vi "InitCSMs.vi"(7 "Enable building lvlibp?":bool, 8 "error in":errorcluster, 11 "testcase-CSMStatus in":refnum<class "testcase-CSMBroadcast.lvclass">) -> (0 "error out":errorcluster, 3 "testcase-CSMStatus out":refnum<class "testcase-CSMBroadcast.lvclass">)   [LabVIEW 2017, in "testcase-CSMBroadcast.lvclass"]
uses:
  testcase-CSMBroadcast.lvclass
  CSM/Normal-CSM.vi
  CSM/Chain1.vi
  CSM/Chain2.vi
  CSM/Chain3.vi
  <vilib>/AppBuilder/AB_API_Simple/Build (path).vi
  CSM/CSM-Testcase.lvlib
  src/user.lib/_NEVSTOP/Communicable State Machine(CSM)/Communicable State Machine.lvlib
  <vilib>/AppBuilder/AB_API_Simple/NI_App_Builder_API.lvlib
panel:
  out "Waited (ms)":u32
  out "CSMs Left":string[](array[string])
  out "CSMs":string[](array[string])
  out "Generated files":path[](array[path])
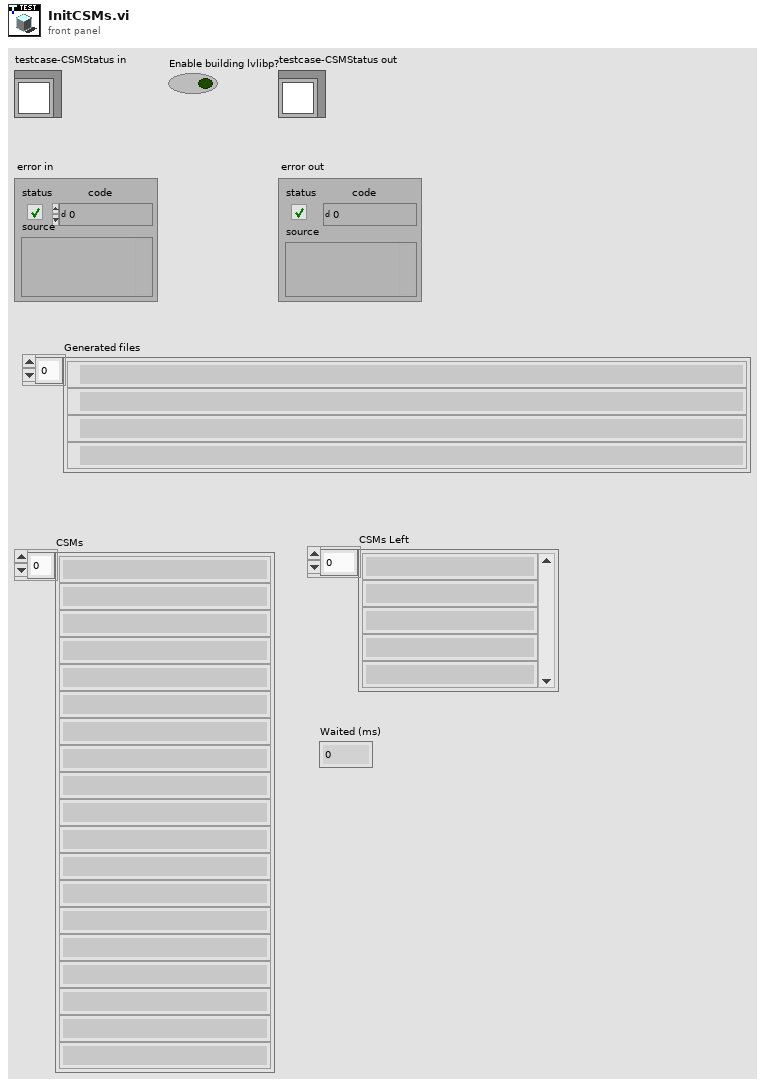
[diagram p1: front panel]
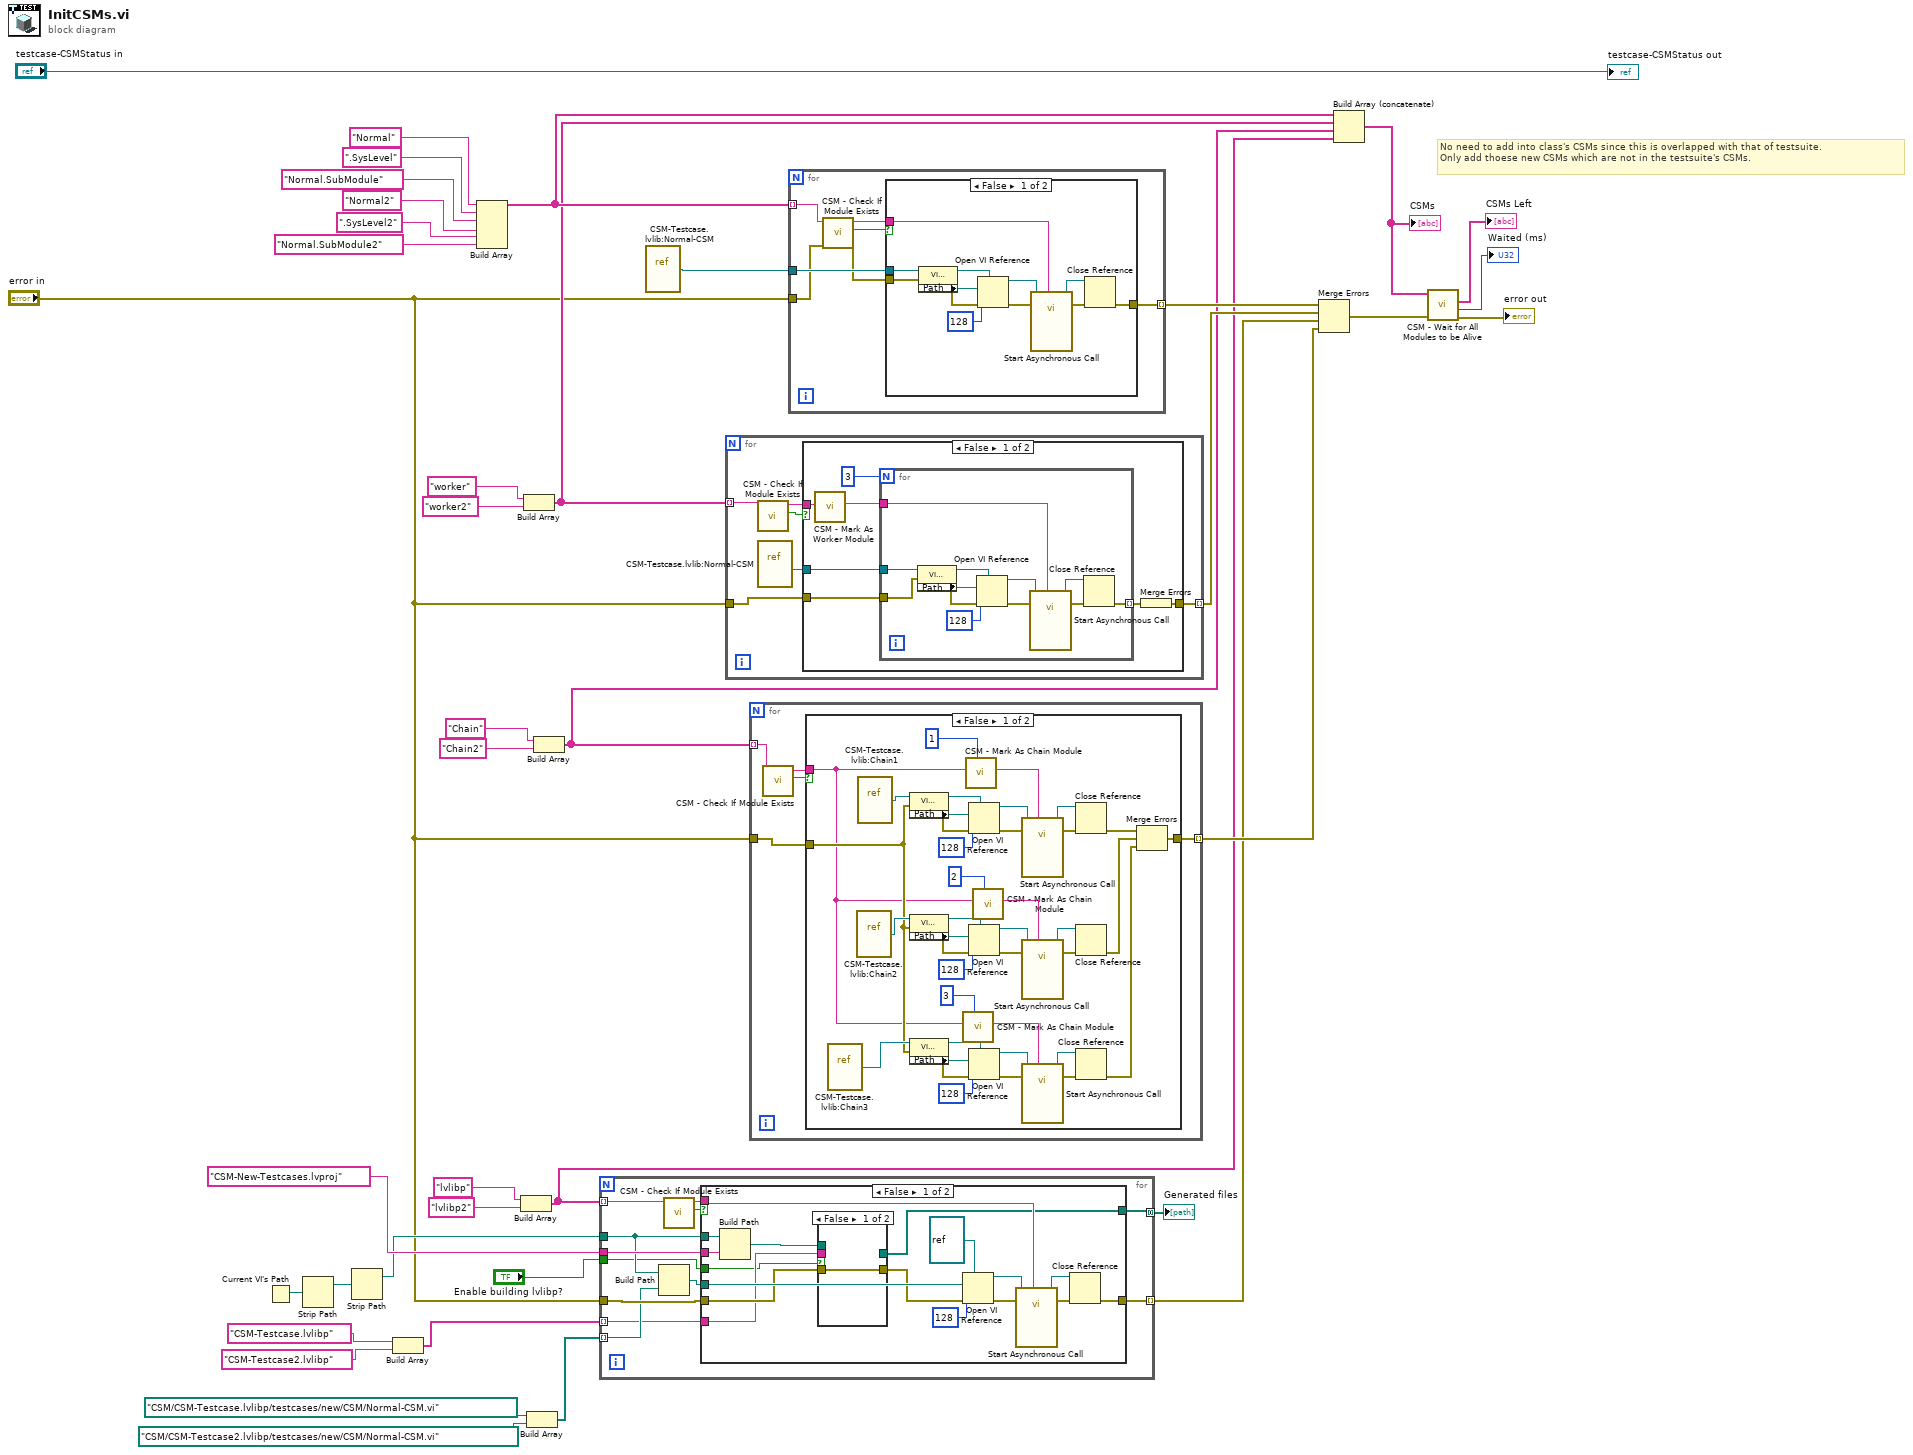
[diagram p0: block diagram]
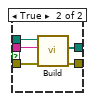
[diagram p2: hidden frame]
diagram:
  # "No need to add into class's CSMs since this is overlapped with that of testsuite.\nOnly add thoese new CSMs which are not in the testsuite's CSMs."
  n1 = Current VI's Path() -> (path=w36:path)
  n2 = Strip Path(path=w36) -> (stripped path=w37:path)  [unwired: 1 out]
  n3 = Strip Path(path=w37) -> (stripped path=w38:path)  [unwired: 1 out]
  n4 = Build Array("CSM-Testcase.lvlibp" ("Name of build specification (if empty: build all)"), "CSM-Testcase2.lvlibp" ("Name of build specification (if empty: build all)")) -> (w10:string[])
  n5 = Build Array("Normal" ("Name (\"\" to Use UUID)"), ".SysLevel" ("Name (\"\" to Use UUID)"), "Normal.SubModule" ("Name (\"\" to Use UUID)"), "Normal2" ("Name (\"\" to Use UUID)"), ".SysLevel2" ("Name (\"\" to Use UUID)"), "Normal.SubModule2" ("Name (\"\" to Use UUID)")) -> (w32:string[])
  n6 = Build Array("lvlibp" ("Name (\"\" to Use UUID)"), "lvlibp2" ("Name (\"\" to Use UUID)")) -> (w16:string[])
  n7 = Build Array("worker" ("Name (\"\" to Use UUID)"), "worker2" ("Name (\"\" to Use UUID)")) -> (w22:string[])
  n8 = Build Array(path "CSM/CSM-Testcase.lvlibp/testcases/new/CSM/Normal-CSM.vi" ("vi path"), path "CSM/CSM-Testcase2.lvlibp/testcases/new/CSM/Normal-CSM.vi" ("vi path")) -> (w13:path[])
  n9 = Build Array("Chain" ("Name (\"\" to Use UUID)"), "Chain2" ("Name (\"\" to Use UUID)")) -> (w19:string[])
  n10 = for {
    tunnel: "CSM-New-Testcases.lvproj" ("name or relative path") -> [w50]
    tunnel: w38 -> [w45]
    tunnel: w16 -> [w47] mode=indexing
    tunnel: w13 -> [w46] mode=indexing
    tunnel: w10 -> [w43] mode=indexing
    tunnel: [w42] -> w9 mode=concatenating
    tunnel: "Enable building lvlibp?" -> [w41]
    tunnel: "error in" -> [w51]
    tunnel: [w49] -> w35 mode=indexing
    n11 = Build Path(base path=w45, name or relative path=w46) -> (appended path=w44:path)
    n12 = call "CSM - Check If Module Exists.vi"("CSM Name"=w47) -> ("Exist?"=w52:bool, "CSM Name (Dup)"=w48:string)  [unwired: 8 in, 1 out]
    n13 = case shown="False" w52 {
      tunnel: [w69 w76] -> w49
      tunnel: w44 -> [w62 _]
      tunnel: w45 -> [w61 _]
      tunnel: w50 -> [w59 _]
      tunnel: w48 -> [w58 _]
      tunnel: w51 -> [w57 w76]
      tunnel: w43 -> [w55 _]
      tunnel: [w54 _] -> w42
      tunnel: w41 -> [w53 _]
      frame False {
        n14 = Build Path(base path=w61, name or relative path=w59) -> (appended path=w60:path)
        n15 = case shown="False" w53 {
          tunnel: w60 -> [_ w75]
          tunnel: w57 -> [w70 w74]
          tunnel: [w70 w73] -> w56
          tunnel: w55 -> [_ w72]
          tunnel: [_ w71] -> w54
          frame False {
          }
          frame True {
            n16 = call-poly <vilib>:"Build.vi"("error in (no error)"=w74, "Name of build specification (if empty: build all)"=w72, "Path to project"=w75) -> ("error out"=w73:errorcluster, "Generated files"=w71:path[])  [unwired: 7 in]
          }
        }
        n17 = Open VI Reference(type specifier VI Refnum (for type only)=refnum<vi> refnum ("reference out"), vi path=w62, options=128, error in (no error)=w56) -> (vi reference=w65:refnum<vi>, error out=w67:errorcluster)  [unwired: 2 in]
        n18 = call-by-ref "Start Asynchronous Call"(reference=w65, error in=w67, "Name (\"\" to Use UUID)"=w58) -> (reference out=w64:refnum<vi>, error out=w66:errorcluster)  [unwired: 11 in]
        n19 = Close Reference(reference=w64, error in (no error)=w66) -> (error out=w69:errorcluster)
      }
      frame True {
      }
    }
  }
  "Generated files" <- w9
  n20 = vi-ref "CSM-Testcase.lvlib:Normal-CSM.vi"() -> (w28:refnum<vi>)
  n21 = for {
    tunnel: w22 -> [w77] mode=indexing
    tunnel: "error in" -> [w82]
    tunnel: [w79] -> w34 mode=indexing
    n22 = call "CSM - Check If Module Exists.vi"("CSM Name"=w77) -> ("Exist?"=w81:bool, "CSM Name (Dup)"=w80:string)  [unwired: 8 in, 1 out]
    n23 = vi-ref "CSM-Testcase.lvlib:Normal-CSM.vi"() -> (w78:refnum<vi>)
    n24 = case shown="False" w81 {
      tunnel: w78 -> [w89 _]
      tunnel: [w83 w102] -> w79
      tunnel: w82 -> [w85 w102]
      tunnel: w80 -> [w84 _]
      frame False {
        n25 = call "CSM - Mark As Worker Module.vi"("CSM Name"=w84) -> ("CSM Name (Marked As Worker)"=w86:string)  [unwired: 9 in]
        n26 = for {
          N: 3 -> [_]
          tunnel: w89 -> [w93]
          tunnel: w86 -> [w92]
          tunnel: [w91] -> w87 mode=indexing
          tunnel: w85 -> [w90]
          n27 = property class="VI (strict)"(reference=w93, error in=w90) -> (reference out=w99:refnum<vi>, error out=w97:errorcluster, "Path"=w96:path)
          n28 = Open VI Reference(type specifier VI Refnum (for type only)=w99, vi path=w96, options=128, error in (no error)=w97) -> (vi reference=w95:refnum<vi>, error out=w100:errorcluster)  [unwired: 2 in]
          n29 = call-by-ref "Start Asynchronous Call"(reference=w95, error in=w100, "Name (\"\" to Use UUID)"=w92) -> (reference out=w94:refnum<vi>, error out=w98:errorcluster)  [unwired: 11 in]
          n30 = Close Reference(reference=w94, error in (no error)=w98) -> (error out=w91:errorcluster)
        }
        n31 = Merge Errors(w87) -> (w83:errorcluster)
      }
      frame True {
      }
    }
  }
  n32 = for {
    tunnel: w19 -> [w103] mode=indexing
    tunnel: "error in" -> [w107]
    tunnel: [w105] -> w40 mode=indexing
    n33 = call "CSM - Check If Module Exists.vi"("CSM Name"=w103) -> ("Exist?"=w106:bool, "CSM Name (Dup)"=w104:string)  [unwired: 8 in, 1 out]
    n34 = case shown="False" w106 {
      tunnel: [w110 w147] -> w105
      tunnel: w107 -> [w109 w147]
      tunnel: w104 -> [w108 _]
      frame False {
        n35 = vi-ref "CSM-Testcase.lvlib:Chain3.vi"() -> (w128:refnum<vi>)
        n36 = vi-ref "CSM-Testcase.lvlib:Chain2.vi"() -> (w129:refnum<vi>)
        n37 = vi-ref "CSM-Testcase.lvlib:Chain1.vi"() -> (w146:refnum<vi>)
        n38 = property class="VI (strict)"(reference=w146, error in=w109) -> (reference out=w143:refnum<vi>, error out=w141:errorcluster, "Path"=w140:path)
        n39 = property class="VI (strict)"(reference=w129, error in=w109) -> (reference out=w132:refnum<vi>, error out=w134:errorcluster, "Path"=w135:path)
        n40 = property class="VI (strict)"(reference=w128, error in=w109) -> (reference out=w125:refnum<vi>, error out=w123:errorcluster, "Path"=w122:path)
        n41 = call "CSM - Mark As Chain Module.vi"("Order"=3, "CSM Name"=w108) -> ("CSM Name (Marked As Chain)"=w116:string)  [unwired: 8 in]
        n42 = call "CSM - Mark As Chain Module.vi"("Order"=1, "CSM Name"=w108) -> ("CSM Name (Marked As Chain)"=w114:string)  [unwired: 8 in]
        n43 = Open VI Reference(type specifier VI Refnum (for type only)=w143, vi path=w140, options=128, error in (no error)=w141) -> (vi reference=w139:refnum<vi>, error out=w144:errorcluster)  [unwired: 2 in]
        n44 = Open VI Reference(type specifier VI Refnum (for type only)=w132, vi path=w135, options=128, error in (no error)=w134) -> (vi reference=w136:refnum<vi>, error out=w131:errorcluster)  [unwired: 2 in]
        n45 = Open VI Reference(type specifier VI Refnum (for type only)=w125, vi path=w122, options=128, error in (no error)=w123) -> (vi reference=w121:refnum<vi>, error out=w126:errorcluster)  [unwired: 2 in]
        n46 = call "CSM - Mark As Chain Module.vi"("Order"=2, "CSM Name"=w108) -> ("CSM Name (Marked As Chain)"=w115:string)  [unwired: 8 in]
        n47 = call-by-ref "Start Asynchronous Call"(reference=w139, error in=w144, "Name (\"\" to Use UUID)"=w114) -> (reference out=w138:refnum<vi>, error out=w142:errorcluster)  [unwired: 11 in]
        n48 = call-by-ref "Start Asynchronous Call"(reference=w136, error in=w131, "Name (\"\" to Use UUID)"=w115) -> (reference out=w137:refnum<vi>, error out=w133:errorcluster)  [unwired: 11 in]
        n49 = call-by-ref "Start Asynchronous Call"(reference=w121, error in=w126, "Name (\"\" to Use UUID)"=w116) -> (reference out=w120:refnum<vi>, error out=w124:errorcluster)  [unwired: 11 in]
        n50 = Close Reference(reference=w138, error in (no error)=w142) -> (error out=w119:errorcluster)
        n51 = Close Reference(reference=w137, error in (no error)=w133) -> (error out=w118:errorcluster)
        n52 = Close Reference(reference=w120, error in (no error)=w124) -> (error out=w117:errorcluster)
        n53 = Merge Errors(w119, w118, w117) -> (w110:errorcluster)
      }
      frame True {
      }
    }
  }
  n54 = for {
    tunnel: w28 -> [w154]
    tunnel: w32 -> [w150] mode=indexing
    tunnel: [w153] -> w33 mode=indexing
    tunnel: "error in" -> [w152]
    n55 = call "CSM - Check If Module Exists.vi"("Error In"=w152, "CSM Name"=w150) -> ("error out"=w151:errorcluster, "Exist?"=w148:bool, "CSM Name (Dup)"=w149:string)  [unwired: 7 in]
    n56 = case shown="False" w148 {
      tunnel: w154 -> [w158 _]
      tunnel: [w157 w167] -> w153
      tunnel: w151 -> [w156 w167]
      tunnel: w149 -> [w155 _]
      frame False {
        n57 = property class="VI (strict)"(reference=w158, error in=w156) -> (reference out=w164:refnum<vi>, error out=w162:errorcluster, "Path"=w161:path)
        n58 = Open VI Reference(type specifier VI Refnum (for type only)=w164, vi path=w161, options=128, error in (no error)=w162) -> (vi reference=w160:refnum<vi>, error out=w165:errorcluster)  [unwired: 2 in]
        n59 = call-by-ref "Start Asynchronous Call"(reference=w160, error in=w165, "Name (\"\" to Use UUID)"=w155) -> (reference out=w159:refnum<vi>, error out=w163:errorcluster)  [unwired: 11 in]
        n60 = Close Reference(reference=w159, error in (no error)=w163) -> (error out=w157:errorcluster)
      }
      frame True {
      }
    }
  }
  n61 = Merge Errors(w33, w34, w35, w40) -> (w7:errorcluster)
  n62 = Build Array (concatenate)(w32, w22, w19, w16) -> (w5:string[])
  "CSMs" <- w5
  n63 = call "CSM - Wait for All Modules to be Alive.vi"("Error In"=w7, "CSM Names"=w5) -> ("error out"=→"error out":errorcluster, "Waited (ms)"=→"Waited (ms)":u32, "CSMs Left"=→"CSMs Left":string[])  [unwired: 7 in]
  "testcase-CSMStatus out" <- "testcase-CSMStatus in"
